vi "tryvi.vi"() -> ()   [LabVIEW 2019]
panel:
  out "subtract":dbl
  out "sum":dbl
  in  "B":dbl
  in  "A":dbl
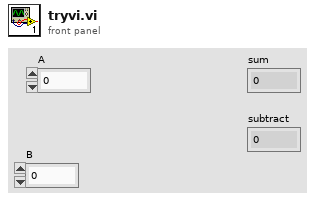
[diagram p1: front panel]
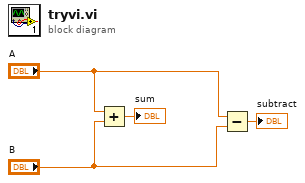
[diagram p0: block diagram]
diagram:
  n1 = Add(x="A", y="B") -> (x+y=→"sum":dbl)
  n2 = Subtract(x="A", y="B") -> (x-y=→"subtract":dbl)
